vi "FlyingDiscShooter_Begin.vi"(8 "error in (no error)":errorcluster) -> (0 "error out":errorcluster)   [LabVIEW 2020]
doc: "Perform initialization actions for the ball shooter system."
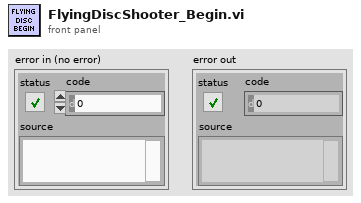
[diagram p1: front panel]
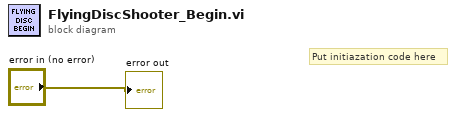
[diagram p0: block diagram]
diagram:
  # "Put initiazation code here"
  "error out" <- "error in (no error)"
